vi "Unit Testing Pump.vi"() -> ()   [LabVIEW 2014]
uses:
  Pump.Simulated class/Pump.Simulated.lvclass
  Pump class/Parameters - cluster.ctl
  Pump class/Pump State - cluster.ctl
  Pump class/Pump.lvclass/Pump.ctl
  <vilib>/JKI/JKI SMO/SMO/Typedefs/SMOState --Enum.ctl
  <vilib>/LabVIEW Open Source Project/Configuration Manager/Manager/Decompose KVPs.vi
  <vilib>/LabVIEW Open Source Project/Configuration Manager/Manager/Write.vi
  <vilib>/LabVIEW Open Source Project/Configuration Manager/Cache/ConfigManager.Cache.lvclass
  <vilib>/JKI/JKI SMO/SMO/SMO.lvclass
  Pump class/Pump.lvclass
  <vilib>/LabVIEW Open Source Project/Configuration Manager/Manager/ConfigManager.lvclass
  <vilib>/addons/_JKI Toolkits/Caraya/classes/Test/Test.lvclass
  <vilib>/addons/_JKI Toolkits/Caraya/classes/Assert/Assert.lvclass
panel:
  out "Pump State":T1(graph)={"Pump Setpoint"=4.754514214207581e-120, "Pump Speed"=6.689422951179204e-230, "Output %"=2.6357709772494154e-160}
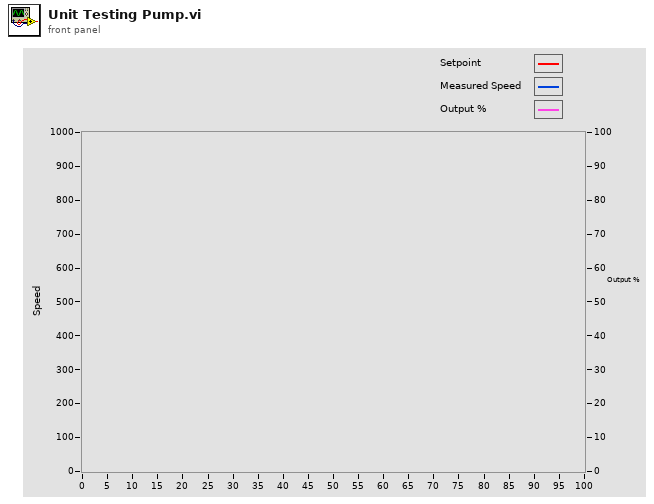
[diagram p1: front panel]
types:
  T1 = typedef "Pump.lvclass/Pump State - cluster.ctl" = cluster{"Pump Setpoint":dbl, "Pump Speed":dbl, "Output %":dbl}
  T2 = typedef "Pump.lvclass/Parameters - cluster.ctl" = cluster{"Kc":dbl, "Ti":dbl, "Td":dbl, "Min Speed":dbl, "Max Speed":dbl}
  T3 = typedef "SMO.lvclass/Public Events.ctl" = cluster{"Error":refnum<user-event>, "State":refnum<user-event>, "Reserve State":refnum<user-event>}
  T4 = typedef "SMO.lvclass/SMOState --Enum.ctl" = enum16{"unknown", "Created", "Started", "Stopped"}
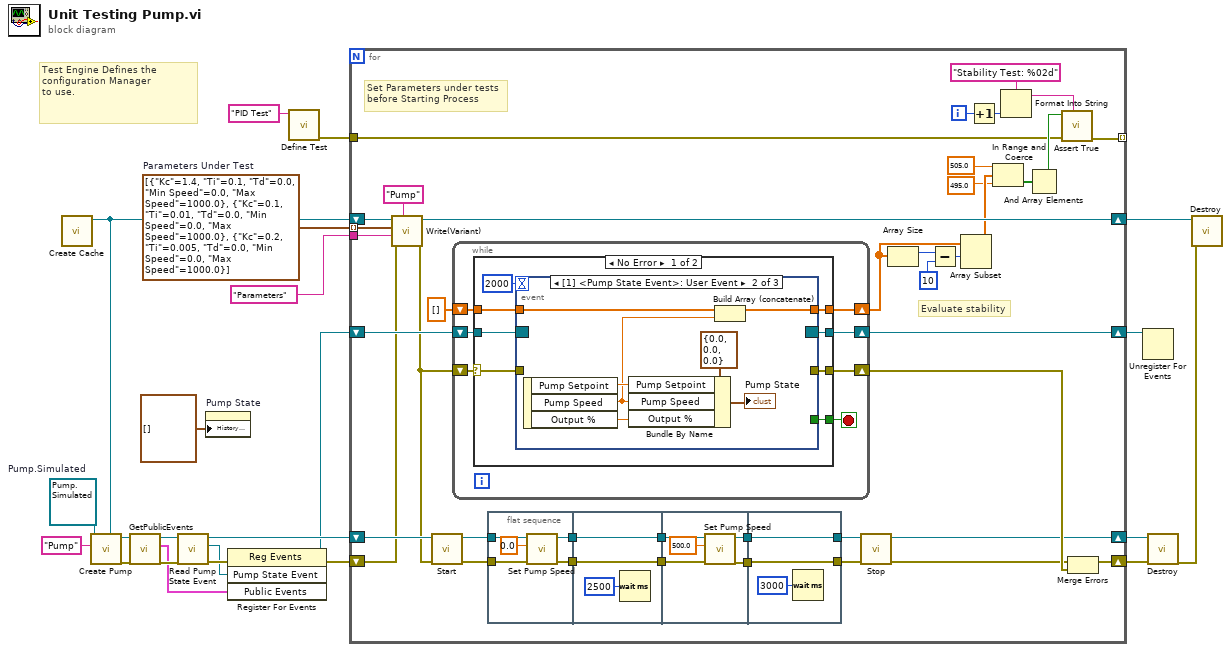
[diagram p0: block diagram]
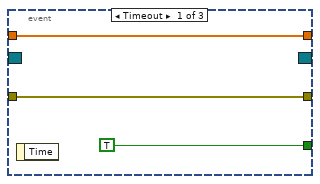
[diagram p2: hidden frame]
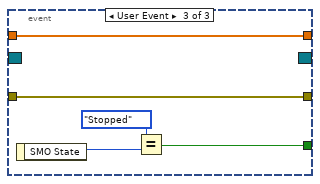
[diagram p3: hidden frame]
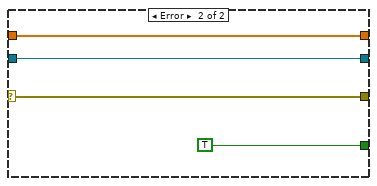
[diagram p4: hidden frame]
diagram:
  w6 = T2[] [{"Kc"=1.4, "Ti"=0.1, "Td"=0.0, "Min Speed"=0.0, "Max Speed"=1000.0}, {"Kc"=0.1, "Ti"=0.01, "Td"=0.0, "Min Speed"=0.0, "Max Speed"=1000.0}, {"Kc"=0.2, "Ti"=0.005, "Td"=0.0, "Min Speed"=0.0, "Max Speed"=1000.0}]  # Parameters Under Test
  w13 = refnum<class "Pump.Simulated.lvclass"> refnum  # Pump.Simulated
  # "Test Engine Defines the configuration Manager\nto use."
  n1 = call <vilib>:"Create Cache.vi"() -> ("ConfigManager.Cache"=w7:refnum<class "ConfigManager.Cache.lvclass">)  [unwired: 11 in]
  n2 = call "Create Pump.vi"("ConfigManager"=w7, "Subsystem Name (Pump)"="Pump", "Pump in"=w13) -> ("error out"=w19:errorcluster, "Pump out"=w21:refnum<class "Pump.Simulated.lvclass">)  [unwired: 6 in, 1 out]
  n3 = call <vilib>:"GetPublicEvents.vi"("error in (no error)"=w19, "SMO"=w21) -> ("error out"=w18:errorcluster, "Public Events"=w17:T3, "SMO out"=w20:refnum<class "Pump.Simulated.lvclass">)  [unwired: 7 in]
  n4 = call "Read Pump State Event.vi"("error in (no error)"=w18, "Pump in"=w20) -> ("error out"=w23:errorcluster, "Pump State Event"=w22:refnum<user-event>, "Pump out"=w16:refnum<class "Pump.Simulated.lvclass">)  [unwired: 7 in]
  n5 = property on="Pump State" class="WFChart (strict)"("History Data"=T1[] []) -> ()  [unwired: 2 in, 2 out]
  n6 = register-events(error in=w23, w22, w17) -> (reference out=w3:refnum<event-registration>, error out=w14:errorcluster)  [unwired: 1 in]
  n7 = call <vilib>:"Define Test.vi"("Label (VI Title)"="PID Test") -> ("error out"=w5:errorcluster)  [unwired: 10 in]
  n8 = for {
    shift-right: [w52] -> w9
    shift-left: w16 -> [w59]
    shift-right: [w58] -> w15
    shift-left: w14 -> [w25]
    shift-right: [w55] -> w11
    shift-left: w7 -> [w47]
    tunnel: w6 -> [w46] mode=indexing
    shift-right: [w40] -> w4
    shift-left: w3 -> [w39]
    tunnel: w5 -> [w27]
    tunnel: [w41] -> _ mode=indexing
    tunnel: "Parameters" ("Subsystem Name (Pump)") -> [w26]
    i -> [w45]
    # "Evaluate stability"
    # "Set Parameters under tests\nbefore Starting Process"
    n9 = call <vilib>:"Write(Variant).vi"("Qualified Name"="Pump" ("Subsystem Name (Pump)"), "error in (no error)"=w25, "Name (empty: value name)"=w26, "value"=w46, "ConfigManager in"=w47) -> ("error out"=w24:errorcluster, "ConfigManager out"=w55:refnum<class "ConfigManager.Cache.lvclass">)  [unwired: 4 in, 1 out]
    n10 = call <vilib>:"Start.vi"("error in (no error)"=w24, "SMO"=w59) -> ("error out"=w53:errorcluster, "SMO out"=w54:refnum<class "Pump.Simulated.lvclass">)  [unwired: 8 in]
    n11 = while {
      shift-right: [w85] -> w40
      shift-left: w39 -> [w86]
      shift-right: [w82] -> w57
      shift-left: w24 -> [w83]
      shift-right: [w80] -> w36
      shift-left: dbl[] [] ("Measured Speed") -> [w81]
      stop <- w84 stop-if-true
      n12 = case shown="No Error" w83 {
        selector: w83 -> [w90 w111]
        tunnel: w86 -> [w93 w113]
        tunnel: [w92 w113] -> w85
        tunnel: [w91 TRUE] -> w84
        tunnel: [w89 w111] -> w82
        tunnel: w81 -> [w88 w110]
        tunnel: [w87 w110] -> w80
        frame No Error {
          n13 = event shown="[1] <Pump State Event>: User Event" {
            selector: w93 -> [_ _ _]
            dyn-events: [_ _ _] -> w92
            timeout: 2000 -> [_ _ _]
            tunnel: [TRUE _ w106] -> w91
            tunnel: w90 -> [w95 _ w109]
            tunnel: [w95 _ w109] -> w89
            tunnel: w88 -> [w96 w101 w105]
            tunnel: [w96 w100 w105] -> w87
            event Timeout {
              n14 = event-data() -> ()  [unwired: 1 in, 1 out]
            }
            event User Event {
              n15 = event-data() -> ("Pump Setpoint"=w103:dbl, "Pump Speed"=w98:dbl, "Output %"=w102:dbl)  [unwired: 1 in]
              n16 = Bundle By Name(cluster=T1 {"Pump Setpoint"=0.0, "Pump Speed"=0.0, "Output %"=0.0} ("Pump State"), "Pump Setpoint"=w103, "Pump Speed"=w98, "Output %"=w102) -> (→"Pump State":T1)
              n17 = Build Array (concatenate)(w101, w98) -> (w100:dbl[])
            }
            event User Event {
              n18 = event-data() -> ("SMO State"=w108:T4)  [unwired: 1 in]
              n19 = Equal?(x=SMOState_--Enum."Stopped", y=w108) -> (x = y?=w106:bool)
            }
          }
        }
        frame Error {
        }
      }
    }
    n20 = flat-sequence {
      tunnel: w53 -> [w65]
      tunnel: w54 -> [w67]
      tunnel: [w66] -> w38
      tunnel: [w64] -> w37
      tunnel: [w71] -> w63
      tunnel: [w70] -> w62
      tunnel: w38 -> [w71]
      tunnel: w37 -> [w70]
      tunnel: [w75] -> w61
      tunnel: [w73] -> w60
      tunnel: w63 -> [w76]
      tunnel: w62 -> [w74]
      tunnel: w61 -> [w79]
      tunnel: w60 -> [w78]
      tunnel: [w79] -> w51
      tunnel: [w78] -> w49
      frame #0 {
        n21 = call "Set Pump Speed.vi"("error in (no error)"=w65, "Speed Command"=0.0, "Pump in"=w67) -> ("error out"=w64:errorcluster, "Pump out"=w66:refnum<class "Pump.Simulated.lvclass">)  [unwired: 5 in, 2 out]
      }
      frame #1 {
        n22 = Wait (ms)(milliseconds to wait=u32 2500) -> ()  [unwired: 1 out]
      }
      frame #2 {
        n23 = call "Set Pump Speed.vi"("error in (no error)"=w74, "Speed Command"=500.0, "Pump in"=w76) -> ("error out"=w73:errorcluster, "Pump out"=w75:refnum<class "Pump.Simulated.lvclass">)  [unwired: 5 in, 2 out]
      }
      frame #3 {
        n24 = Wait (ms)(milliseconds to wait=u32 3000) -> ()  [unwired: 1 out]
      }
    }
    n25 = call <vilib>:"Stop.vi"("error in (no error)"=w49, "SMO"=w51) -> ("error out"=w50:errorcluster, "SMO out"=w52:refnum<class "Pump.Simulated.lvclass">)  [unwired: 8 in]
    n26 = Array Size(array=w36) -> (size(s)=w35:i32)
    n27 = Subtract(x=w35, y=10 ("length")) -> (x-y=w33:i32)
    n28 = Array Subset(array=w36, index=w33) -> (w32:dbl[])  [unwired: 1 in]
    n29 = Increment(x=w45) -> (x+1=w42:i32)
    n30 = In Range and Coerce(upper limit=505.0 ("Speed Command"), x=w32, lower limit=495.0 ("Speed Command")) -> (In Range?=w31:bool[])  [unwired: 1 out]
    n31 = Format Into String(format string="Stability Test: %02d", w42) -> (resulting string=w43:string)  [unwired: 2 in, 1 out]
    n32 = And Array Elements(Boolean array=w31) -> (logical AND=w30:bool)
    n33 = call <vilib>:"Assert True.vi"("Label"=w43, "error in (no error)"=w27, "True?"=w30) -> ("error out"=w41:errorcluster)  [unwired: 8 in]
    n34 = Merge Errors(w50, w57) -> (w58:errorcluster)
  }
  n35 = Unregister For Events(event registration refnum=w4) -> ()  [unwired: 1 in, 1 out]
  n36 = call <vilib>:"Destroy.vi"("error in (no error)"=w15, "SMO"=w9) -> ("error out"=w10:errorcluster)  [unwired: 9 in]
  n37 = call-dynamic <vilib>:"Destroy.vi"("error in (no error)"=w10, "ConfigManager.Cache in"=w11) -> ()  [unwired: 8 in, 2 out]
